vi "运维调试_其他.vi"() -> ()   [LabVIEW 2016, in "其他.lvlib"]
uses:
  <vilib>/Utility/miscctls.llb/LVPointTypeDef.ctl
panel:
  in  "隐藏按钮":bool
  out "TCP接收全局簇":T1={"网络灯"=FALSE, "接收中"=TRUE, "已接收百分比"="", "接收成功次数"=0.0}
  out "TCP发送全局簇":T2={"网络灯"=FALSE, "发送中"=TRUE, "已发送百分比"="", "发送成功次数"=0.0}
  out "传输次数":dbl
types:
  T1 = cluster{"网络灯":bool, "接收中":bool, "已接收百分比":string, "接收成功次数":dbl}
  T2 = cluster{"网络灯":bool, "发送中":bool, "已发送百分比":string, "发送成功次数":dbl}
  T3 = typedef "LVPointTypeDef.ctl" = cluster{"Horizontal":i16, "Vertical":i16}
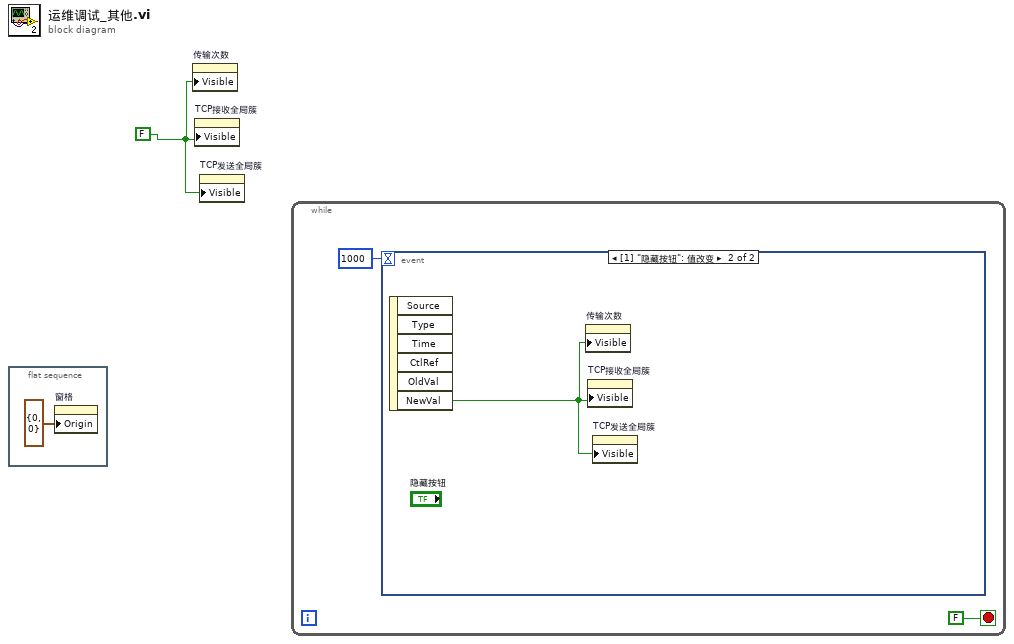
[diagram p0: block diagram]
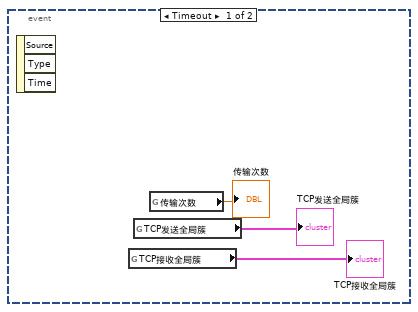
[diagram p2: hidden frame]
diagram:
  w1 = FALSE
  n1 = flat-sequence {
    frame #0 {
      n2 = property on="窗格" class="Pane"("Origin"=T3 {"Horizontal"=0, "Vertical"=0} ("原点")) -> ()  [unwired: 2 in, 2 out]
    }
  }
  n3 = property on="传输次数" class="DigNum (严格)"("Visible"=w1) -> ()  [unwired: 2 in, 2 out]
  n4 = property on="TCP接收全局簇" class="Clust (严格)"("Visible"=w1) -> ()  [unwired: 2 in, 2 out]
  n5 = property on="TCP发送全局簇" class="Clust (严格)"("Visible"=w1) -> ()  [unwired: 2 in, 2 out]
  n6 = while {
    stop <- FALSE stop-if-true
    n7 = event shown="[1] \"隐藏按钮\": 值改变" {
      selector: _ -> [_ _]
      dyn-events: _ -> [_ _]
      timeout: 1000 -> [_ _]
      event Timeout {
        n8 = event-data() -> ()  [unwired: 1 in, 3 out]
        n9 = global read "全局变量1.vi" "TCP接收全局簇"() -> (→"TCP接收全局簇":T1)
        n10 = global read "全局变量1.vi" "TCP发送全局簇"() -> (→"TCP发送全局簇":T2)
        n11 = global read "全局变量1.vi" "传输次数"() -> (→"传输次数":dbl)
      }
      event "隐藏按钮": Value Change {
        n12 = event-data() -> ("NewVal"=w8:bool)  [unwired: 1 in, 5 out]
        n13 = property on="传输次数" class="DigNum (严格)"("Visible"=w8) -> ()  [unwired: 2 in, 2 out]
        n14 = property on="TCP接收全局簇" class="Clust (严格)"("Visible"=w8) -> ()  [unwired: 2 in, 2 out]
        n15 = property on="TCP发送全局簇" class="Clust (严格)"("Visible"=w8) -> ()  [unwired: 2 in, 2 out]
      }
    }
  }
